vi "needRamp.vi"(11 "AMI_Cluster":T1) -> (3 "needRamp?":bool)   [LabVIEW 2019]
uses:
  Monitor Communication/AMI/AMI_cluster.ctl
panel:
  # "AMI-Cluster"
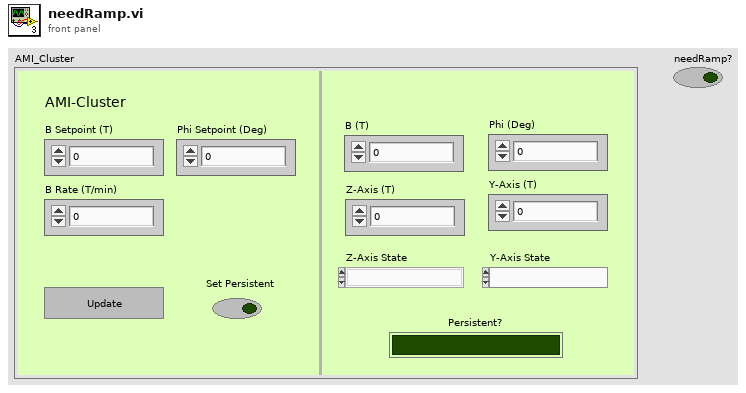
[diagram p1: front panel]
types:
  T1 = typedef "AMI_cluster.ctl" = cluster{"Set Persistent":bool, "B (T)":dbl, "B Setpoint (T)":dbl, "Phi (Deg)":dbl, "Phi Setpoint (Deg)":dbl, "B Rate (T/min)":dbl, "Y-Axis (T)":dbl, "Z-Axis (T)":dbl, "Z-Axis State":enum16{"", "RAMPING", "HOLDING", "PAUSED", "MANUAL UP", "MANUAL DOWN", "ZEROING CURRENT", "QUENCH DETECTED", "AT ZERO", "HEATING SWITCH", "COOLING SWITCH", "EXTERNAL RAMPDOWN"}, "Y-Axis State":enum16{"", "RAMPING", "HOLDING", "PAUSED", "MANUAL UP", "MANUAL DOWN", "ZEROING CURRENT", "QUENCH DETECTED", "AT ZERO", "HEATING SWITCH", "COOLING SWITCH", "EXTERNAL RAMPDOWN"}, "Update":bool, "Persistent?":bool}
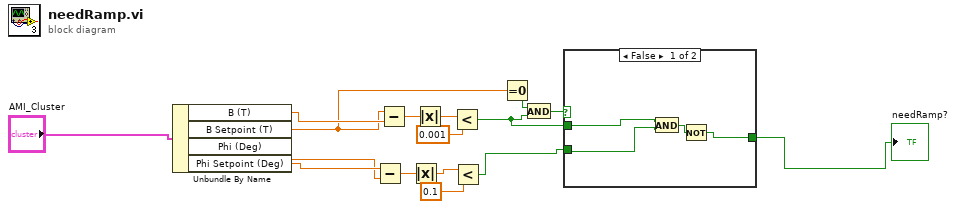
[diagram p0: block diagram]
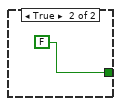
[diagram p2: hidden frame]
diagram:
  n1 = Unbundle By Name("AMI_Cluster") -> ("B (T)"=w7:dbl, "B Setpoint (T)"=w6:dbl, "Phi (Deg)"=w12:dbl, "Phi Setpoint (Deg)"=w13:dbl)
  n2 = Subtract(x=w13, y=w12) -> (x-y=w14:dbl)
  n3 = Subtract(x=w6, y=w7) -> (x-y=w10:dbl)
  n4 = Absolute Value(x=w14) -> (abs(x)=w15:dbl)
  n5 = Absolute Value(x=w10) -> (abs(x)=w9:dbl)
  n6 = Less?(x=w9, y=0.001) -> (x < y?=w1:bool)
  n7 = Less?(x=w15, y=0.1) -> (x < y?=w2:bool)
  n8 = Equal To 0?(x=w6) -> (x = 0?=w5:bool)
  n9 = And(x=w5, y=w1) -> (x .and. y?=w4:bool)
  n10 = case shown="False" w4 {
    tunnel: [w20 FALSE] -> w3
    tunnel: w2 -> [w18 _]
    tunnel: w1 -> [w19 _]
    frame False {
      n11 = And(x=w19, y=w18) -> (x .and. y?=w17:bool)
      n12 = Not(x=w17) -> (.not. x?=w20:bool)
    }
    frame True {
    }
  }
  "needRamp?" <- w3
